vi "TEST_r_w_L1.vi"() -> ()   [LabVIEW 2012]
panel:
  in  "Combination":i32 min=0 max=127 step=1 format="%b"
  in  "Single/Comb":bool=TRUE
  in  "Single Channel Enable":i32(slide) scale=0.0..6.0
  out "error out":errorcluster
  out "data read value":u32=36
  in  "Data":i32
  in  "Register or channel":i32=96
  out "data out serial":string="0_2-63@36\r\n"
  in  "RD/#WR":bool
  in  "error in (no error)":errorcluster
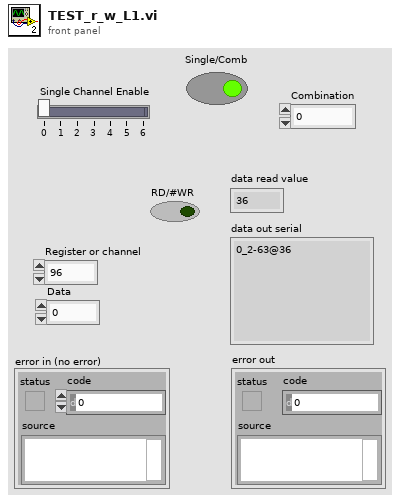
[diagram p1: front panel]
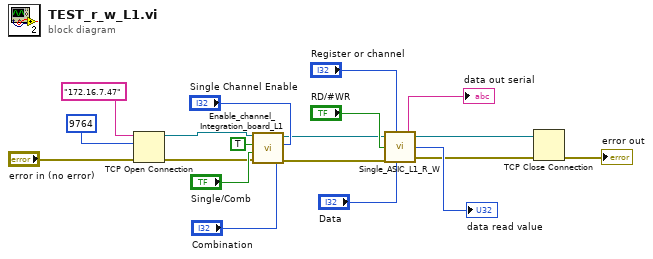
[diagram p0: block diagram]
diagram:
  n1 = TCP Open Connection(address="172.16.7.47", remote port or service name=9764, error in (no error)="error in (no error)") -> (connection ID=w2:refnum<k5>, error out=w4:errorcluster)  [unwired: 2 in]
  n2 = call "Enable_channel_Integration_board_L1.vi"("Cobination"="Combination", "Enable  L1 single  Input"="Single Channel Enable", "error in (no error)"=w4, "SingleIN/#Combination"="Single/Comb", "#Enable all L1"=TRUE, "connection ID"=w2) -> ("error out"=w3:errorcluster, "connection ID out"=w1:refnum<k5>)
  n3 = call "Single_ASIC_L1_R_W.vi"("connection ID"=w1, "Register or channel"="Register or channel", "RD/#WR"="RD/#WR", "error in (no error)"=w3, "Data"="Data") -> ("data out serial"=→"data out serial":string, "connection ID out"=w9:refnum<k5>, "data read value"=→"data read value":u32, "error out"=w10:errorcluster)  [unwired: 1 in]
  n4 = TCP Close Connection(connection ID=w9, error in (no error)=w10) -> (error out=→"error out":errorcluster)  [unwired: 1 in, 1 out]
